vi "item_OnCommand.vi"(10 "Command ID":string, 11 "Object":T1) -> ()   [LabVIEW 2019, in "BlueSerializationProvider.lvlib"]
uses:
  BlueSerializationProvider.lvlib
  <resource>/Framework/Providers/API/ItemRef.ctl
  <vilib>/Utility/error.llb/DialogType.ctl
  BlueSerializationScripts/BlueSerializationScripts.lvlib
panel:
  out "error out":errorcluster
  in  "error in":errorcluster
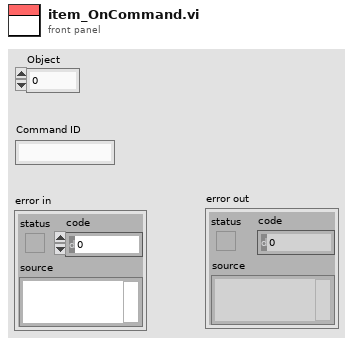
[diagram p1: front panel]
types:
  T1 = typedef "ItemRef.ctl" = u64
  T2 = typedef "DialogType.ctl" = u16
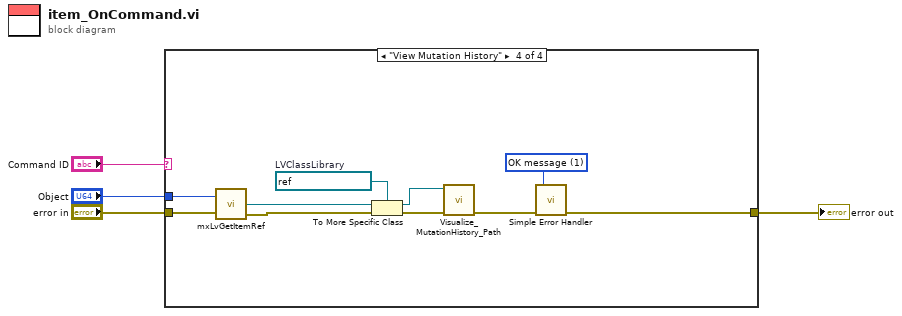
[diagram p0: block diagram]
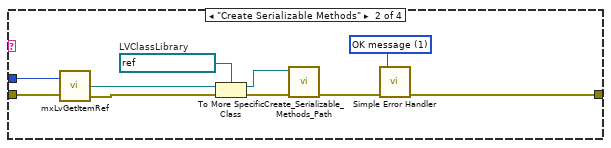
[diagram p3: hidden frame]
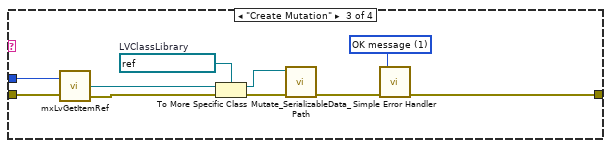
[diagram p4: hidden frame]
diagram:
  n1 = case shown="\"View Mutation History\"" "Command ID" {
    tunnel: "Object" -> [_ w8 w21 w31]
    tunnel: "error in" -> [w5 w7 w20 w30]
    tunnel: [w5 w6 w19 w29] -> w1
    frame Default {
    }
    frame "Create Serializable Methods" {
      w12 = T2 1 items=["no dialog", "OK message", "continue or stop message", "OK message + warnings", "continue/stop + warnings"] ("type of dialog (OK msg:1)")
      w15 = refnum<vi> refnum  # LVClassLibrary
      n2 = call <resource>:"mxLvGetItemRef.vi"("Item"=w8, "error in"=w7) -> ("Item Refnum"=w14:refnum<vi>, "error out"=w13:errorcluster)  [unwired: 1 out]
      n3 = To More Specific Class(target class=w15, reference=w14, error in=w13) -> (specific class reference=w9:refnum<vi>, error out=w10:errorcluster)
      n4 = call "Create_Serializable_Methods_Path.vi"("error in (no error)"=w10, "class reference"=w9) -> ("error out"=w11:errorcluster)  [unwired: 9 in]
      n5 = call <vilib>:"Simple Error Handler.vi"("type of dialog (OK msg:1)"=w12, "error in (no error)"=w11) -> ("error out"=w6:errorcluster)  [unwired: 3 in, 4 out]
    }
    frame "Create Mutation" {
      w22 = T2 1 items=["no dialog", "OK message", "continue or stop message", "OK message + warnings", "continue/stop + warnings"] ("type of dialog (OK msg:1)")
      w25 = refnum<vi> refnum  # LVClassLibrary
      n6 = call <resource>:"mxLvGetItemRef.vi"("Item"=w21, "error in"=w20) -> ("Item Refnum"=w24:refnum<vi>, "error out"=w23:errorcluster)  [unwired: 1 out]
      n7 = To More Specific Class(target class=w25, reference=w24, error in=w23) -> (specific class reference=w16:refnum<vi>, error out=w18:errorcluster)
      n8 = call "Mutate_SerializableData_Path.vi"("error in (no error)"=w18, "class reference"=w16) -> ("error out"=w17:errorcluster)  [unwired: 9 in]
      n9 = call <vilib>:"Simple Error Handler.vi"("type of dialog (OK msg:1)"=w22, "error in (no error)"=w17) -> ("error out"=w19:errorcluster)  [unwired: 3 in, 4 out]
    }
    frame "View Mutation History" {
      w32 = T2 1 items=["no dialog", "OK message", "continue or stop message", "OK message + warnings", "continue/stop + warnings"] ("type of dialog (OK msg:1)")
      w35 = refnum<vi> refnum  # LVClassLibrary
      n10 = call <resource>:"mxLvGetItemRef.vi"("Item"=w31, "error in"=w30) -> ("Item Refnum"=w34:refnum<vi>, "error out"=w33:errorcluster)  [unwired: 1 out]
      n11 = To More Specific Class(target class=w35, reference=w34, error in=w33) -> (specific class reference=w28:refnum<vi>, error out=w27:errorcluster)
      n12 = call "Visualize_MutationHistory_Path.vi"("error in (no error)"=w27, "class reference"=w28) -> ("error out"=w26:errorcluster)  [unwired: 9 in]
      n13 = call <vilib>:"Simple Error Handler.vi"("type of dialog (OK msg:1)"=w32, "error in (no error)"=w26) -> ("error out"=w29:errorcluster)  [unwired: 3 in, 4 out]
    }
  }
  "error out" <- w1
